vi "svx_Polar_Draw_IndicationArcsBG.vi"(4 "shaft rotating direction":u16, 6 "probe angle [deg]":u16, 7 "Background color":u32, 8 "grid measurements":T2={"pixel center"={"x"=0, "y"=0}, "scale factors"={"a"=0.0, "b"=0.0, "log?(F)"=FALSE}, "grid color"=16860, "start angle"=0.0, "end angle"=360.0, "tick length"=0, "pixel radius"=0} {"end angle" format="%0.2f"; "start angle" format="%0.2f"; "scale factors"."b" format="%0.2f"; "scale factors"."a" format="%0.2f"}, 9 "Indication Arcs":T1, 10 "width/max":dbl, 11 "Picture":picture) -> (3 "new picture":picture)   [LabVIEW 2017, in "SVX Polar Plot.xctl"]
uses:
  <vilib>/addons/_XControls/Polar Plot/SVX Polar Plot.xctl
  <vilib>/addons/_XControls/Polar Plot/subVIs/svx_Polar_Indication_Arcs.ctl
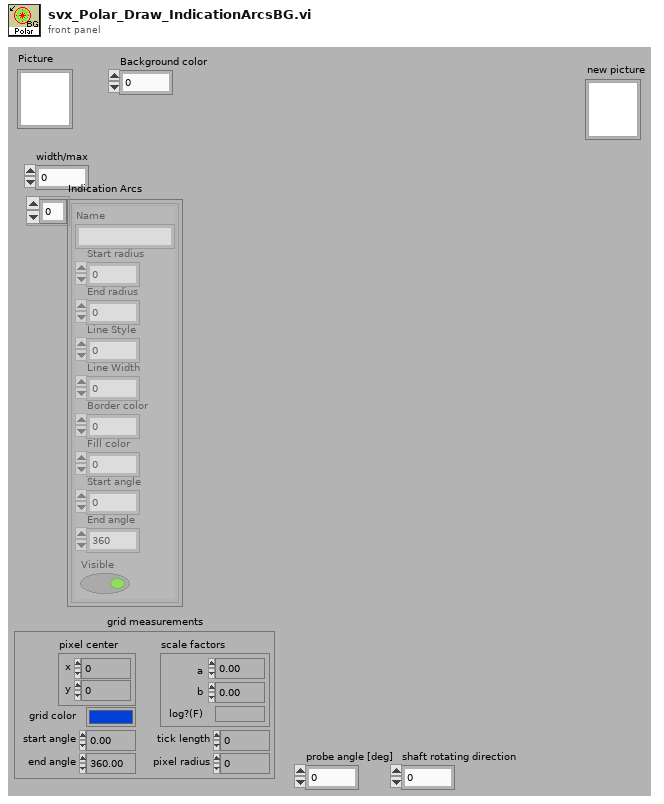
[diagram p1: front panel]
types:
  T1 = typedef "SVX Polar Plot.xctl/svx_Polar_Indication_Arcs.ctl" = cluster{"Name":string, "Start radius":dbl, "End radius":dbl, "Line Style":i32, "Line Width":i32, "Border color":u32, "Fill color":u32, "Start angle":i16, "End angle":i16, "Visible":bool}[]
  T2 = cluster{"pixel center":cluster{"x":i16, "y":i16}, "scale factors":cluster{"a":dbl, "b":dbl, "log?(F)":bool}, "grid color":u32, "start angle":dbl, "end angle":dbl, "tick length":i16, "pixel radius":i32}
  T3 = cluster{"Width":u16, "Style":enum32{"Solid", "Dash", "Dot", "DashDot", "DashDotDot"}}
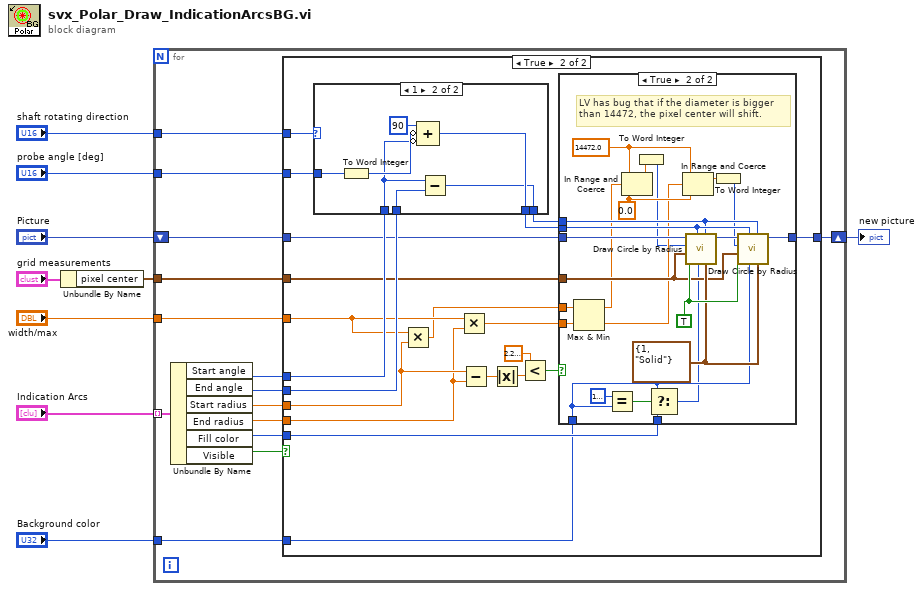
[diagram p0: block diagram]
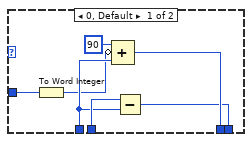
[diagram p4: hidden frame]
diagram:
  n1 = Unbundle By Name("grid measurements") -> ("pixel center"=w6:cluster{"x":i16, "y":i16})
  n2 = for {
    tunnel: "Indication Arcs" -> [w23] mode=indexing
    tunnel: "width/max" -> [w22]
    tunnel: w6 -> [w21]
    shift-right: [w19] -> w5
    shift-left: "Picture" -> [w20]
    tunnel: "shaft rotating direction" -> [w16]
    tunnel: "probe angle [deg]" -> [w17]
    tunnel: "Background color" -> [w12]
    n3 = Unbundle By Name(w23) -> ("Start angle"=w18:i16, "End angle"=w10:i16, "Start radius"=w11:dbl, "End radius"=w14:dbl, "Fill color"=w13:u32, "Visible"=w15:bool)
    n4 = case shown="True" w15 {
      tunnel: w11 -> [_ w34]
      tunnel: w22 -> [_ w40]
      tunnel: w21 -> [_ w36]
      tunnel: w20 -> [w24 w25]
      tunnel: [w24 w39] -> w19
      tunnel: w10 -> [_ w44]
      tunnel: w18 -> [_ w43]
      tunnel: w17 -> [_ w42]
      tunnel: w16 -> [_ w41]
      tunnel: w14 -> [_ w33]
      tunnel: w13 -> [_ w27]
      tunnel: w12 -> [_ w26]
      frame False {
      }
      frame True {
        n5 = case shown="1" w41 {
          tunnel: [w74 w81] -> w38
          tunnel: w44 -> [w73 w76]
          tunnel: w43 -> [w72 w77]
          tunnel: [w71 w80] -> w37
          tunnel: w42 -> [w70 w79]
          frame 0, Default {
            n6 = To Word Integer(number=w70) -> (16bit integer=w69:i16)
            n7 = Compound Arithmetic op=ADD(i16 90 ("value"), invert w69, w72) -> (w74:i16)
            n8 = Subtract(x=w73, y=w72) -> (x-y=w71:i16)
          }
          frame 1 {
            n9 = To Word Integer(number=w79) -> (16bit integer=w78:i16)
            n10 = Compound Arithmetic op=ADD(i16 90 ("value"), invert w78, invert w77) -> (w81:i16)
            n11 = Subtract(x=w77, y=w76) -> (x-y=w80:i16)
          }
        }
        n12 = Multiply(x=w40, y=w34) -> (x*y=w28:dbl)
        n13 = Multiply(x=w40, y=w33) -> (x*y=w35:dbl)
        n14 = Subtract(x=w34, y=w33) -> (x-y=w32:dbl)
        n15 = Absolute Value(x=w32) -> (abs(x)=w31:dbl)
        n16 = Less?(x=2.220446049250313e-16, y=w31) -> (x < y?=w29:bool)
        n17 = case shown="True" w29 {
          tunnel: w25 -> [w45 w56]
          tunnel: [w45 w57] -> w39
          tunnel: w38 -> [_ w67]
          tunnel: w37 -> [_ w66]
          tunnel: w36 -> [_ w63]
          tunnel: w35 -> [_ w54]
          tunnel: w28 -> [_ w55]
          tunnel: w27 -> [_ w59]
          tunnel: w26 -> [_ w60]
          frame False {
          }
          frame True {
            w51 = 0.0 ("lower limit")
            w52 = 14472.0 ("upper limit")
            w65 = TRUE ("fill?(F)")
            w64 = T3 {"Width"=1, "Style"=enum."Solid"} ("pen")
            # "LV has bug that if the diameter is bigger\nthan 14472, the pixel center will shift."
            n18 = Max & Min(x=w55, y=w54) -> (max(x,y)=w53:dbl, min(x,y)=w50:dbl)
            n19 = Equal?(x=u32 16777216, y=w60) -> (x = y?=w61:bool)
            n20 = In Range and Coerce(upper limit=w52, x=w53, lower limit=w51) -> (coerced(x)=w47:dbl)  [unwired: 1 out]
            n21 = To Word Integer(number=w47) -> (16bit integer=w46:i16)
            n22 = Select(t=w60, s=w61, f=w59) -> (s? t:f=w58:u32)
            n23 = In Range and Coerce(upper limit=w52, x=w50, lower limit=w51) -> (coerced(x)=w49:dbl)  [unwired: 1 out]
            n24 = call <vilib>:"Draw Circle by Radius.vi"("pen"=w64, "arc size(360)"=w66, "color(black)"=w58, "start angle(0)"=w67, "fill?(F)"=w65, "pixel center"=w63, "radius"=w46, "picture"=w56) -> ("new picture"=w68:picture)  [unwired: 3 in]
            n25 = To Word Integer(number=w49) -> (16bit integer=w48:i16)
            n26 = call <vilib>:"Draw Circle by Radius.vi"("pen"=w64, "arc size(360)"=w66, "color(black)"=w60, "start angle(0)"=w67, "fill?(F)"=w65, "pixel center"=w63, "radius"=w48, "picture"=w68) -> ("new picture"=w57:picture)  [unwired: 3 in]
          }
        }
      }
    }
  }
  "new picture" <- w5
